vi "Traccia_Vin_Vout_2015led.vi"() -> ()   [LabVIEW 2014]
doc: "Traccia_Vin_Vout\nUtilizza Vin_Vout e traccia una curva Vout vs Vin\n9/2011, 9/2015 vers. LV2014 \nFM & ADL"
uses:
  <vilib>/Utility/file.llb/Write To Spreadsheet File (DBL).vi
panel:
  in  "Scala Asse Y":enum8{"Lineare", "Logaritmica"}(ring)
  in  "R (kOhm)":dbl=2.2 min=-10.0 max=10.0 step=0.1 format="%_4g"
  in  "Fondo Scala AI0":dbl(ring)=10.0 items=["10"=10.0, "5"=5.0, "0.5"=0.5, "0.05"=0.05]
  in  "SALVA I DATI SU FILE":bool=TRUE caption="ON\nOFF"
  out "N. misura":i16
  out "Corrente in funzione della tensione ai capi":cluster{dbl[], dbl[]}(graph)
  out "Vin (V)":dbl format="%_4g"
  out "Vout (V)":dbl format="%_4f"
  in  "Numero misure":i16=10 min=0 max=1000 step=1
  in  "Vmax(V)x":dbl=5.0 min=-10.0 max=10.0 step=0.1 format="%_4g"
  in  "Vmin(V)":dbl=-5.0 min=-10.0 max=10.0 step=0.1 format="%_4g"
  # "1) Scegliere il fondo scala dell'analog input: \n[10, 5, 0.5, 0.05]"
  # "Collegare il CB 22 (analog output) all'ingresso Vin  \ne il CB68 all'uscita Vout . \nLa terra del circuito (CB29) DEVE essere in comune alla terra della scheda."
  # "2) Selezionare il valore minimo e massimo della tensione di ingresso ed il numero di valori \n(equispaziati  tra gli estremi)"
  # "3) Premere la freccia bianca"
  # "Durante la misura gli indicatori  mostrano i valori di Vin e Vout ed il numero progressivo della misura"
  # "Sul grafico viene mostrata la tensione di uscita in funzione della tensione di ingresso."
  # "NO\nSI"
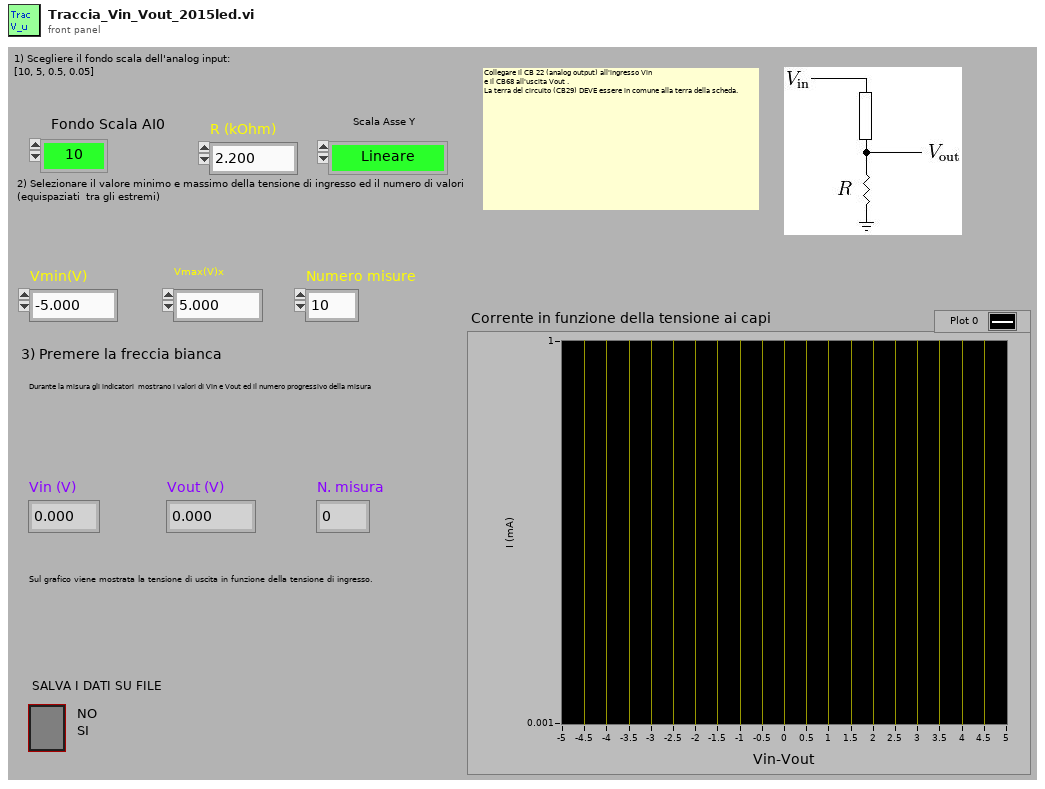
[diagram p1: front panel]
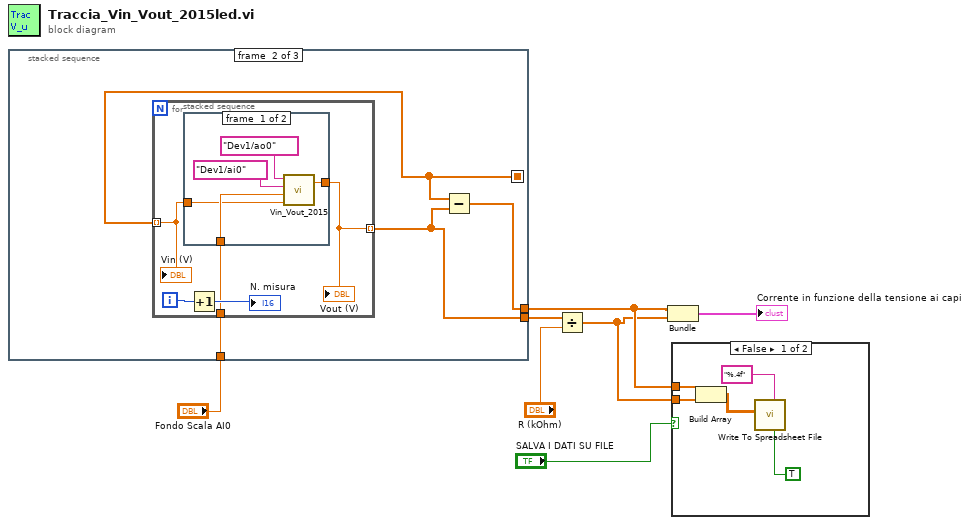
[diagram p0: block diagram]
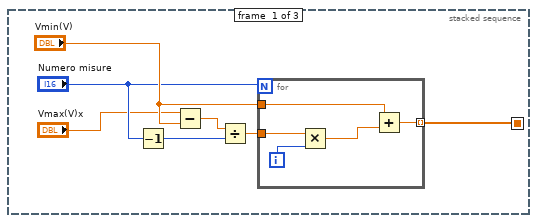
[diagram p3: hidden frame]
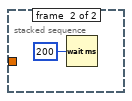
[diagram p4: hidden frame]
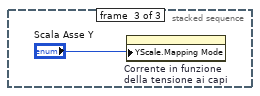
[diagram p5: hidden frame]
diagram:
  n1 = stacked-sequence {
    seq-local: [w10 _ _] -> [_ w22 _]
    tunnel: [_ w21 _] -> w2
    tunnel: [_ w20 _] -> w6
    tunnel: "Fondo Scala AI0" -> [_ w23 _]
    frame #0 {
      n2 = Decrement(x="Numero misure") -> (x-1=w13:i16)
      n3 = Subtract(x="Vmax(V)x", y="Vmin(V)") -> (x-y=w14:dbl)
      n4 = Divide(x=w14, y=w13) -> (x/y=w12:dbl)
      n5 = for {
        N: "Numero misure" -> [_]
        tunnel: "Vmin(V)" -> [w19]
        tunnel: [w18] -> w10 mode=indexing
        tunnel: w12 -> [w17]
        i -> [w16]
        n6 = Multiply(x=w17, y=w16) -> (x*y=w15:dbl)
        n7 = Add(x=w19, y=w15) -> (x+y=w18:dbl)
      }
    }
    frame #1 {
      n8 = for {
        tunnel: w22 -> [w28] mode=indexing
        tunnel: [w27] -> w21 mode=indexing
        tunnel: w23 -> [w24]
        i -> [w26]
        n9 = stacked-sequence {
          tunnel: w28 -> [w31 _]
          tunnel: [w33 _] -> w27
          tunnel: w24 -> [w32 _]
          frame #0 {
            n10 = call "Vin_Vout_2015.vi"("V in volt"=w31, "Fondo Scala 6024"=w32, "Canale Ingresso"=tag "Dev1/ai0", "Canale uscita"=tag "Dev1/ao0") -> ("mean Vout"=w33:dbl)  [unwired: 1 out]
          }
          frame #1 {
            n11 = Wait (ms)(milliseconds to wait=u32 200) -> ()  [unwired: 1 out]
          }
        }
        "Vout (V)" <- w27
        n12 = Increment(x=w26) -> (x+1=→"N. misura":i32)
        "Vin (V)" <- w28
      }
      n13 = Subtract(x=w22, y=w21) -> (x-y=w20:dbl[])
    }
    frame #2 {
      n14 = property on="Corrente in funzione della tensione ai capi" class="XYGraph (strict)"("YScale.Mapping Mode"="Scala Asse Y") -> ()  [unwired: 2 in, 2 out]
    }
  }
  n15 = Divide(x=w2, y="R (kOhm)") -> (x/y=w3:dbl[])
  n16 = Bundle(w6, w3) -> (→"Corrente in funzione della tensione ai capi":cluster{dbl[], dbl[]})  [unwired: 1 in]
  n17 = case shown="False" "SALVA I DATI SU FILE" {
    tunnel: w3 -> [w40 _]
    tunnel: w6 -> [w39 _]
    frame False {
      n18 = Build Array(w39, w40) -> (w38:dbl[][])
      n19 = call-poly <vilib>:"Write To Spreadsheet File.vi"("transpose? (no:F)"=TRUE, "format (%.3f)"="%.4f", "2D data"=w38) -> ()  [unwired: 5 in, 1 out]
    }
    frame True {
    }
  }
